vi "distance 2 stop at 0.vi"(10 "speed":dbl) -> (2 "Distance":dbl)   [LabVIEW 2017]
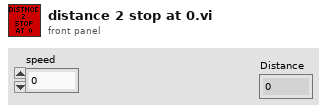
[diagram p1: front panel]
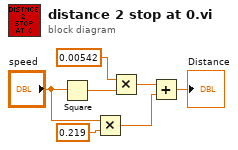
[diagram p0: block diagram]
diagram:
  n1 = Square(x="speed") -> (x^2=w5:dbl)
  n2 = Multiply(x="speed", y=0.219) -> (x*y=w3:dbl)
  n3 = Multiply(x=0.00542, y=w5) -> (x*y=w2:dbl)
  n4 = Add(x=w2, y=w3) -> (x+y=→"Distance":dbl)
